vi "Mandelbrot.vi"() -> ()   [LabVIEW 2019, in "Mandelbrot.lvlib"]
uses:
  Mandelbrot.lvlib
  subVIs/app_event.ctl
  subVIs/axis_info.ctl
panel:
  out "render time (s)":dbl format="%<%H:%M:%S%3u>t"
  in  "colors":string(combo)="jet"
  in  "Julia root":cdb=-0.75+0.25i
  in  "fractal selector":enum16{"Mandelbrot", "Julia"}(ring)
  in  "reset buttom":bool
  in  "max iterations":u32=75
  out "Intensity Graph":i32[][](graph)
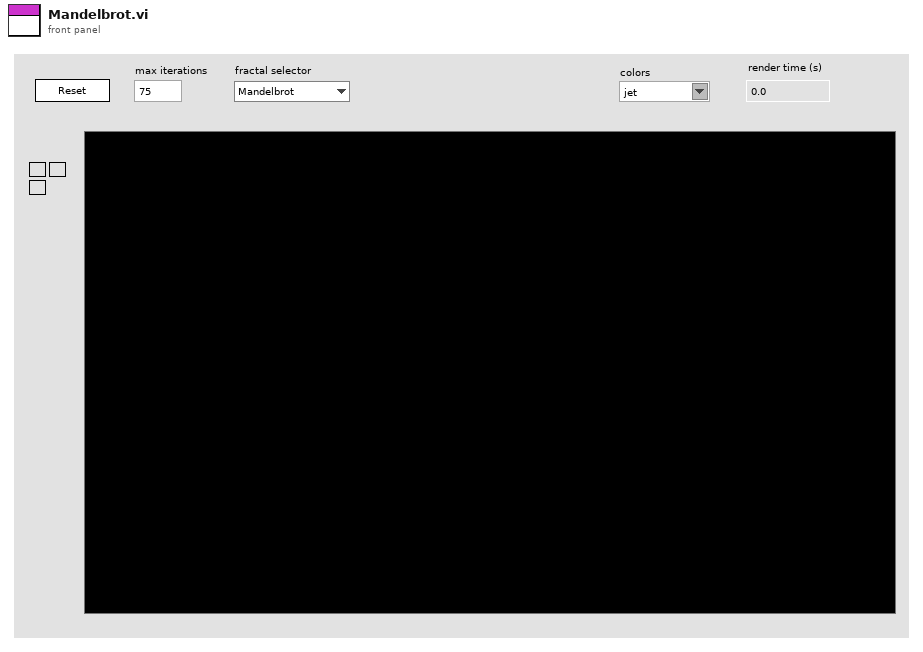
[diagram p1: front panel]
types:
  T1 = typedef "Mandelbrot.lvlib/app_event.ctl" = enum16{"initialize", "refresh", "shutdown", "exit"}
  T2 = typedef "Mandelbrot.lvlib/axis_info.ctl" = cluster{"samples":u32, "end":dbl, "start":dbl}
  T3 = typedef "LVOffsetAndMultiplierTypeDef.ctl" = cluster{"Offset":dbl, "Multiplier":dbl}
  T4 = enum32{"invalid app kind", "Development System", "Run Time System", "Student Edition", "Embedded LabVIEW", "Evaluation", "Custom"}
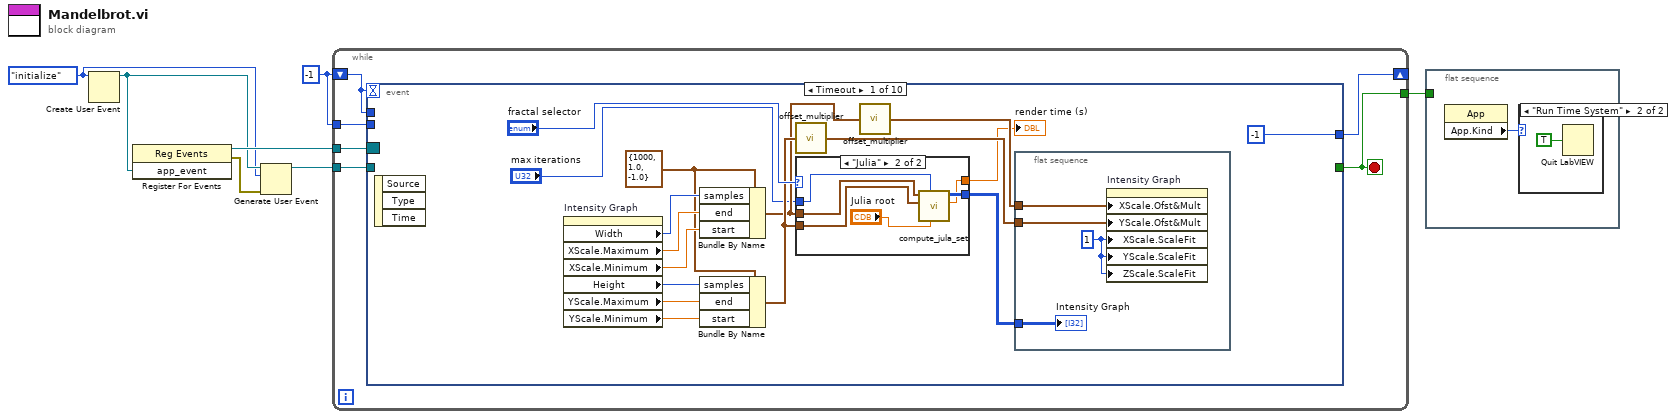
[diagram p0: block diagram]
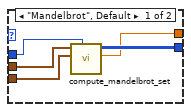
[diagram p3: hidden frame]
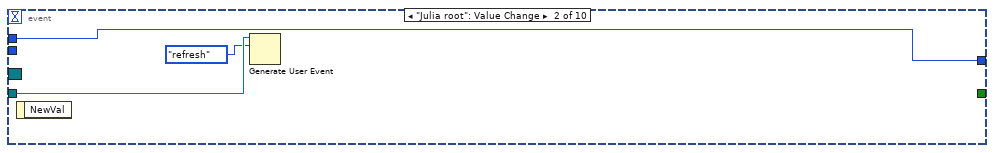
[diagram p4: hidden frame]
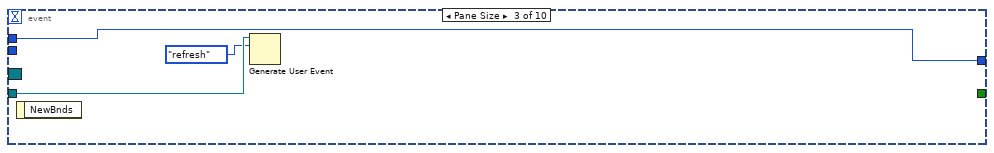
[diagram p5: hidden frame]
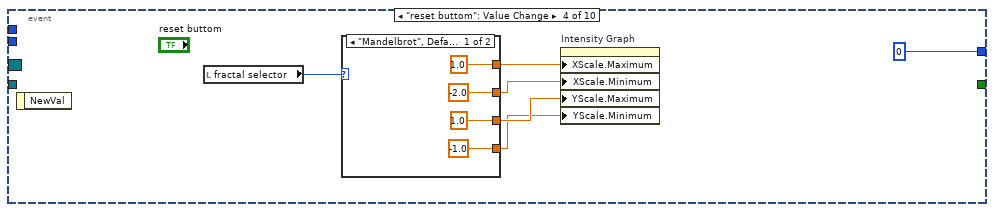
[diagram p6: hidden frame]
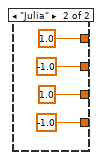
[diagram p7: hidden frame]
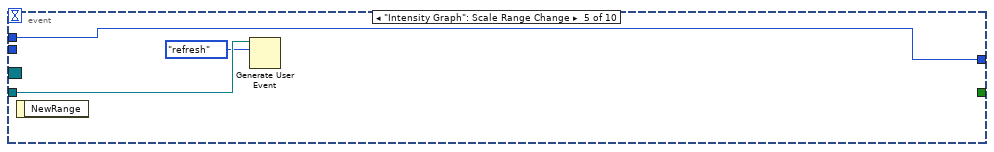
[diagram p8: hidden frame]
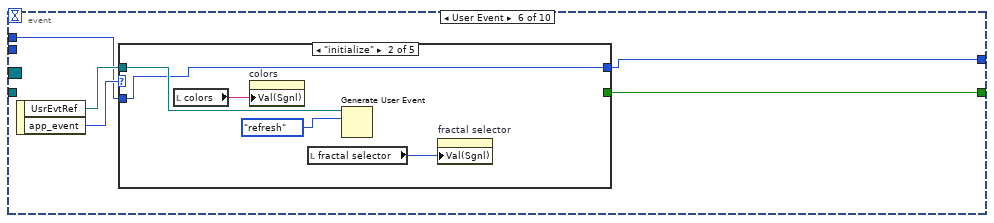
[diagram p9: hidden frame]
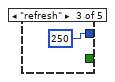
[diagram p11: hidden frame]
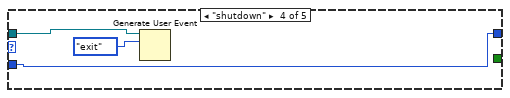
[diagram p12: hidden frame]
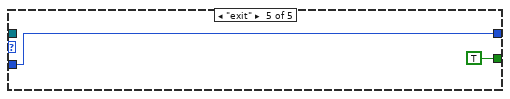
[diagram p13: hidden frame]
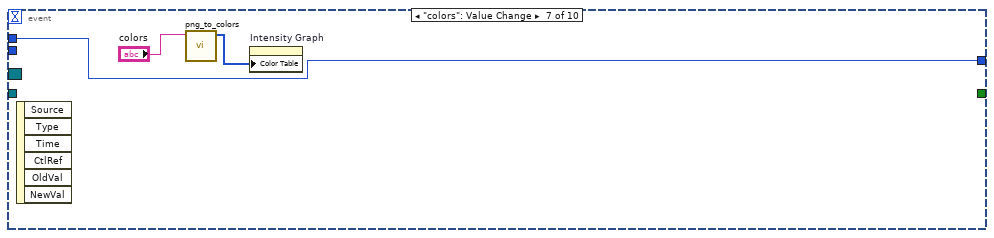
[diagram p14: hidden frame]
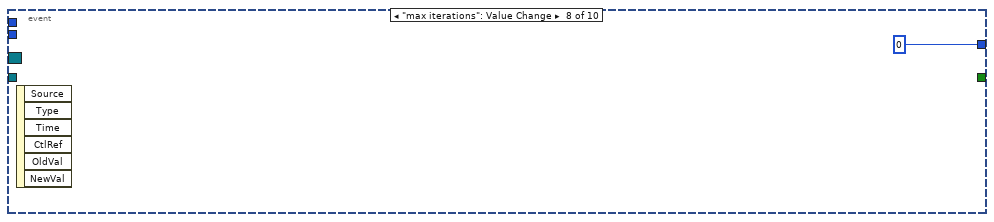
[diagram p15: hidden frame]
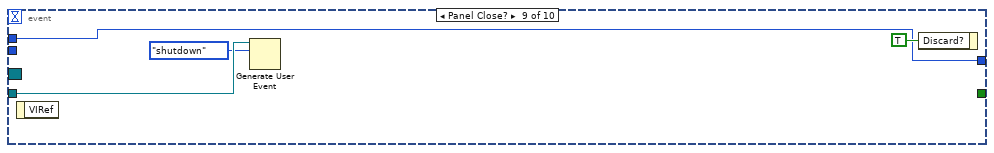
[diagram p16: hidden frame]
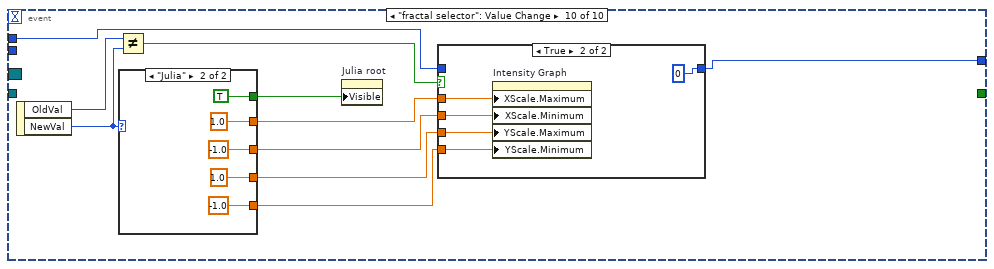
[diagram p17: hidden frame]
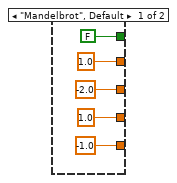
[diagram p19: hidden frame]
diagram:
  w3 = -1
  w4 = app_event."initialize" ("app_event")
  n1 = Create User Event(user event datatype=w4) -> (user event=w5:refnum<user-event>)  [unwired: 1 in, 1 out]
  n2 = register-events(w5) -> (reference out=w7:refnum<event-registration>, error out=w6:errorcluster)  [unwired: 2 in]
  n3 = Generate User Event(user event=w5, event data cluster=w4, error in=w6) -> (user event out=w2:refnum<user-event>)  [unwired: 1 in, 1 out]
  n4 = while {
    tunnel: w7 -> [w13]
    shift-right: [w11] -> _
    shift-left: w3 -> [w8]
    tunnel: w3 -> [w12]
    tunnel: w2 -> [w10]
    tunnel: [w9] -> w1
    stop <- w9 stop-if-true
    n5 = event shown="[0] Timeout" {
      selector: w13 -> [_ _ _ _ _ _ _ _ _ _]
      dyn-events: _ -> [_ _ _ _ _ _ _ _ _ _]
      timeout: w8 -> [_ _ _ _ _ _ _ _ _ _]
      tunnel: w12 -> [_ _ _ _ _ _ _ _ _ _]
      tunnel: [-1 w45 w48 0 w65 w70 w85 0 w89 w101] -> w11
      tunnel: [_ _ _ _ _ w69 _ _ _ _] -> w9
      tunnel: w10 -> [_ w47 w50 _ w67 _ _ _ w91 _]
      tunnel: w8 -> [_ w45 w48 _ w65 w68 w85 _ w89 w93]
      event Timeout {
        w21 = T2 {"samples"=1000, "end"=1.0, "start"=-1.0} ("x axis")
        n6 = event-data() -> ()  [unwired: 1 in, 3 out]
        n7 = property on="Intensity Graph" class="IntGraph (strict)"() -> ("Width"=w27:u32, "XScale.Maximum"=w26:dbl, "XScale.Minimum"=w25:dbl, "Height"=w24:u32, "YScale.Maximum"=w23:dbl, "YScale.Minimum"=w22:dbl)  [unwired: 2 in, 2 out]
        n8 = Bundle By Name(cluster=w21, "samples"=w27, "end"=w26, "start"=w25) -> (w19:T2)
        n9 = Bundle By Name(cluster=w21, "samples"=w24, "end"=w23, "start"=w22) -> (w20:T2)
        n10 = call "offset_multiplier.vi"("axis info"=w20) -> ("offset & multiplier"=w17:T3)
        n11 = case shown="\"Julia\"" "fractal selector" {
          tunnel: w19 -> [w38 w44]
          tunnel: w20 -> [w37 w43]
          tunnel: [w36 w42] -> w14
          tunnel: "max iterations" -> [w35 w40]
          tunnel: [w34 w39] -> w15
          frame "Mandelbrot", Default {
            n12 = call "compute_mandelbrot_set.vi"("max iter"=w35, "y axis"=w37, "x axis"=w38) -> ("render time"=w34:dbl, "fractal set"=w36:i32[][])  [unwired: 7 in]
          }
          frame "Julia" {
            n13 = call "compute_jula_set.vi"("x + iy"="Julia root", "max iter"=w40, "y axis"=w43, "x axis"=w44) -> ("render time"=w39:dbl, "fractal set"=w42:i32[][])  [unwired: 6 in]
          }
        }
        "render time (s)" <- w15
        n14 = call "offset_multiplier.vi"("axis info"=w19) -> ("offset & multiplier"=w18:T3)
        n15 = flat-sequence {
          tunnel: w14 -> [w31]
          tunnel: w18 -> [w33]
          tunnel: w17 -> [w32]
          frame #0 {
            w30 = u8 1 ("X Scale.Scale Fit")
            n16 = property on="Intensity Graph" class="IntGraph (strict)"("XScale.Ofst&Mult"=w33, "YScale.Ofst&Mult"=w32, "XScale.ScaleFit"=w30, "YScale.ScaleFit"=w30, "ZScale.ScaleFit"=w30) -> ()  [unwired: 2 in, 2 out]
            "Intensity Graph" <- w31
          }
        }
      }
      event "Julia root": Value Change {
        n17 = event-data() -> ()  [unwired: 1 in, 1 out]
        n18 = Generate User Event(user event=w47, event data cluster=app_event."refresh" ("event data")) -> ()  [unwired: 2 in, 2 out]
      }
      event Pane Size {
        n19 = event-data() -> ()  [unwired: 1 in, 1 out]
        n20 = Generate User Event(user event=w50, event data cluster=app_event."refresh" ("event data")) -> ()  [unwired: 2 in, 2 out]
      }
      event "reset buttom": Value Change {
        n21 = event-data() -> ()  [unwired: 1 in, 1 out]
        n22 = local read "fractal selector"() -> (w55:enum16{"Mandelbrot", "Julia"})
        n23 = case shown="\"Mandelbrot\", Default" w55 {
          tunnel: [-1.0 ("Y Scale.Range:Minimum") -1.0 ("Y Scale.Range:Minimum")] -> w51
          tunnel: [1.0 ("Y Scale.Range:Maximum") 1.0 ("Y Scale.Range:Maximum")] -> w52
          tunnel: [-2.0 ("X Scale.Range:Minimum") -1.0 ("X Scale.Range:Minimum")] -> w53
          tunnel: [1.0 ("X Scale.Range:Maximum") 1.0 ("X Scale.Range:Maximum")] -> w54
          frame "Mandelbrot", Default {
          }
          frame "Julia" {
          }
        }
        n24 = property on="Intensity Graph" class="IntGraph (strict)"("XScale.Maximum"=w54, "XScale.Minimum"=w53, "YScale.Maximum"=w52, "YScale.Minimum"=w51) -> ()  [unwired: 2 in, 2 out]
      }
      event "Intensity Graph": Scale Range Change {
        n25 = event-data() -> ()  [unwired: 1 in, 1 out]
        n26 = Generate User Event(user event=w67, event data cluster=app_event."refresh" ("event data")) -> ()  [unwired: 2 in, 2 out]
      }
      event User Event {
        n27 = event-data() -> ("UsrEvtRef"=w71:refnum<user-event>, "app_event"=w72:T1)  [unwired: 1 in]
        n28 = case shown="\"initialize\"" w72 {
          tunnel: w71 -> [_ w78 _ w81 _]
          tunnel: [w73 w76 250 w82 w84] -> w70
          tunnel: w68 -> [w73 w76 _ w82 w84]
          tunnel: [_ _ _ _ TRUE] -> w69
          frame Default {
          }
          frame "initialize" {
            n29 = local read "colors"() -> (w74:string)
            n30 = property on="colors" class="CmbBox"("Val(Sgnl)"=w74) -> ()  [unwired: 2 in, 2 out]
            n31 = local read "fractal selector"() -> (w75:enum16{"Mandelbrot", "Julia"})
            n32 = Generate User Event(user event=w78, event data cluster=app_event."refresh" ("event data")) -> ()  [unwired: 2 in, 2 out]
            n33 = property on="fractal selector" class="Enum (strict)"("Val(Sgnl)"=w75) -> ()  [unwired: 2 in, 2 out]
          }
          frame "refresh" {
          }
          frame "shutdown" {
            n34 = Generate User Event(user event=w81, event data cluster=app_event."exit" ("event data")) -> ()  [unwired: 2 in, 2 out]
          }
          frame "exit" {
          }
        }
      }
      event "colors": Value Change {
        n35 = event-data() -> ()  [unwired: 1 in, 6 out]
        n36 = call "png_to_colors.vi"("colors"="colors") -> ("colors"=w87:u32[])  [unwired: 10 in]
        n37 = property on="Intensity Graph" class="IntGraph (strict)"("Color Table"=w87) -> ()  [unwired: 2 in, 2 out]
      }
      event "max iterations": Value Change {
        n38 = event-data() -> ()  [unwired: 1 in, 6 out]
      }
      event Panel Close? {
        n39 = event-data() -> ()  [unwired: 1 in, 1 out]
        n40 = Generate User Event(user event=w91, event data cluster=app_event."shutdown" ("event data")) -> ()  [unwired: 2 in, 2 out]
        n41 = event-data("Discard?"=TRUE) -> ()  [unwired: 1 in, 1 out]
      }
      event "fractal selector": Value Change {
        n42 = event-data() -> ("OldVal"=w96:enum16{"Mandelbrot", "Julia"}, "NewVal"=w95:enum16{"Mandelbrot", "Julia"})  [unwired: 1 in]
        n43 = Not Equal?(x=w96, y=w95) -> (x != y?=w94:bool)
        n44 = case shown="\"Julia\"" w95 {
          tunnel: [FALSE TRUE] -> w102
          tunnel: [-1.0 ("Y Scale.Range:Minimum") -1.0 ("Y Scale.Range:Minimum")] -> w100
          tunnel: [1.0 ("Y Scale.Range:Maximum") 1.0 ("Y Scale.Range:Maximum")] -> w99
          tunnel: [-2.0 ("X Scale.Range:Minimum") -1.0 ("X Scale.Range:Minimum")] -> w98
          tunnel: [1.0 ("X Scale.Range:Maximum") 1.0 ("X Scale.Range:Maximum")] -> w97
          frame "Mandelbrot", Default {
          }
          frame "Julia" {
          }
        }
        n45 = property on="Julia root" class="DigNum (strict)"("Visible"=w102) -> ()  [unwired: 2 in, 2 out]
        n46 = case shown="True" w94 {
          tunnel: [w103 0] -> w101
          tunnel: w100 -> [_ w107]
          tunnel: w99 -> [_ w106]
          tunnel: w98 -> [_ w105]
          tunnel: w97 -> [_ w104]
          tunnel: w93 -> [w103 _]
          frame False {
          }
          frame True {
            n47 = property on="Intensity Graph" class="IntGraph (strict)"("XScale.Maximum"=w104, "XScale.Minimum"=w105, "YScale.Maximum"=w106, "YScale.Minimum"=w107) -> ()  [unwired: 2 in, 2 out]
          }
        }
      }
    }
  }
  n48 = flat-sequence {
    tunnel: w1 -> [_]
    frame #0 {
      n49 = property class="App"() -> ("App.Kind"=w119:T4)  [unwired: 2 in, 2 out]
      n50 = case shown="\"Run Time System\"" w119 {
        frame Default {
        }
        frame "Run Time System" {
          n51 = Quit LabVIEW(quit? (T)=TRUE) -> ()
        }
      }
    }
  }
